vi "Add 1.vi"() -> ()   [LabVIEW 2019]
panel:
  out "Slide":u8(slide) scale=0.0..100.0
  in  "Boolean":bool
  in  "b":dbl
  in  "a":dbl
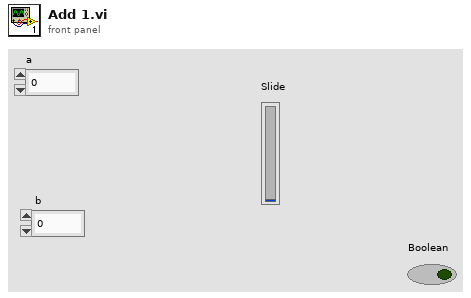
[diagram p1: front panel]
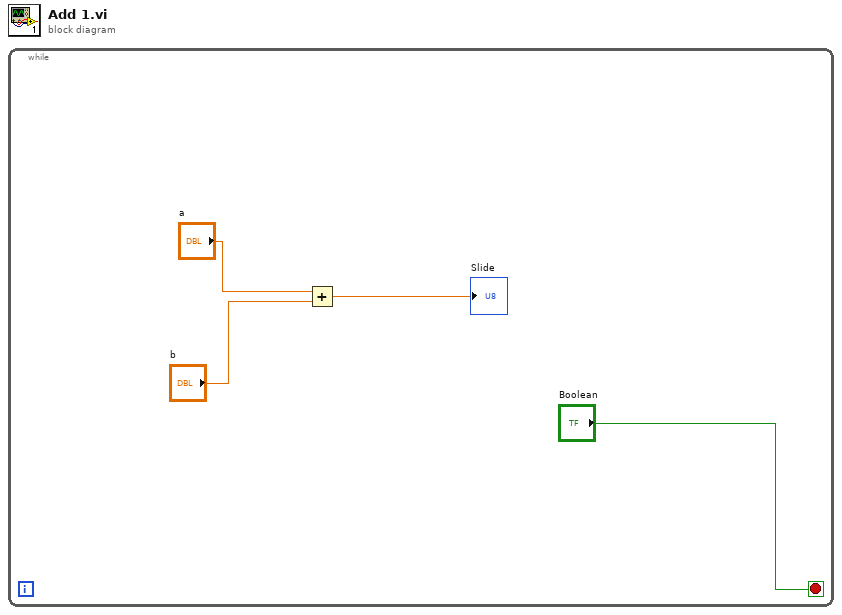
[diagram p0: block diagram]
diagram:
  n1 = while {
    stop <- "Boolean" stop-if-true
    n2 = Add(x="a", y="b") -> (x+y=→"Slide":dbl)
  }
